vi "3D-DataCollect.vi"(0 "Barcode":string, 1 "USLandLSL":cluster{"USL":dbl, "LSL":dbl}[](array[cluster]), 2 "Max Value":string[][](array[string]), 3 "LabelArray":string[](array[string]), 4 "Date Message":string[](array[string])) -> (14 "ResultNumberMessage":string[][](array[string]), 15 "ResultNumber":i32[](array[numeric]))   [LabVIEW 2015]
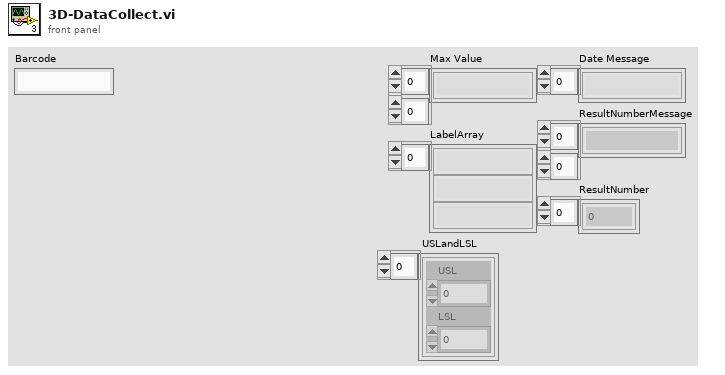
[diagram p1: front panel]
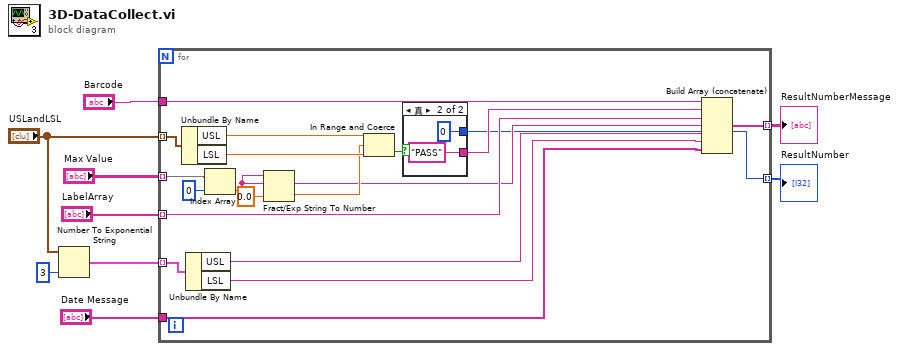
[diagram p0: block diagram]
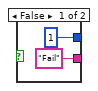
[diagram p2: hidden frame]
diagram:
  n1 = Number To Exponential String(number="USLandLSL", precision (6)=i16 3 ("精度(6)")) -> (E-format string=w4:cluster{"USL":string, "LSL":string}[])  [unwired: 2 in]
  n2 = for {
    tunnel: "Max Value" -> [w23] mode=indexing
    tunnel: "LabelArray" -> [w17] mode=indexing
    tunnel: "USLandLSL" -> [w26] mode=indexing
    tunnel: "Date Message" -> [w12]
    tunnel: "Barcode" -> [w27]
    tunnel: w4 -> [w15] mode=indexing
    tunnel: [w11] -> w2 mode=indexing
    tunnel: [w10] -> w1 mode=indexing
    n3 = Unbundle By Name(w26) -> ("USL"=w25:dbl, "LSL"=w24:dbl)
    n4 = Unbundle By Name(w15) -> ("USL"=w14:string, "LSL"=w13:string)
    n5 = Index Array(array=w23, index=0 ("索引")) -> (element=w16:string)
    n6 = Fract/Exp String To Number(string=w16, default (0 dbl)=0.0 ("默认(0 DBL)")) -> (number=w20:dbl)  [unwired: 2 in, 1 out]
    n7 = In Range and Coerce(upper limit=w25, x=w20, lower limit=w24) -> (In Range?=w19:bool)  [unwired: 1 out]
    n8 = case shown="真" w19 {
      tunnel: ["Fail" "PASS"] -> w18
      tunnel: [1 0] -> w10
      frame False {
      }
      frame True {
      }
    }
    n9 = Build Array (concatenate)(w27, w18, w17, w16, w14, w13, w12) -> (w11:string[])
  }
  "ResultNumberMessage" <- w2
  "ResultNumber" <- w1
